vi "InterTrial.vi"(8 "error in (no error)":errorcluster, 11 "TrialBasedExperiment in":refnum<class "MatlabExperiment.lvclass">) -> (0 "error out":errorcluster, 2 "Timeout":dbl, 3 "TrialBasedExperiment out":refnum<class "MatlabExperiment.lvclass">)   [LabVIEW 2010, in "MatlabExperiment.lvclass"]
uses:
  MatlabExperiment.lvclass
  TrialBasedExperimentObject/TrialBasedExperiment.lvclass
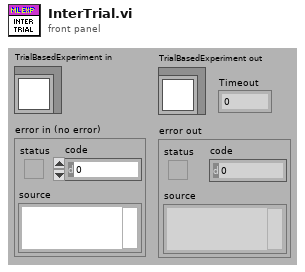
[diagram p1: front panel]
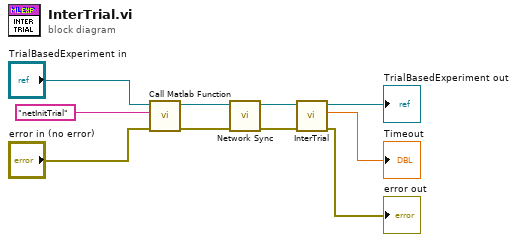
[diagram p0: block diagram]
diagram:
  n1 = call-dynamic "Call Matlab Function.vi"("error in (no error)"="error in (no error)", "Function name"="netInitTrial", "TrialBasedExperiment in"="TrialBasedExperiment in") -> ("error out"=w3:errorcluster, "TrialBasedExperiment out"=w4:refnum<class "MatlabExperiment.lvclass">)  [unwired: 5 in, 2 out]
  n2 = call "Network Sync.vi"("error in (no error)"=w3, "MatlabExperiment in"=w4) -> ("error out"=w2:errorcluster, "MatlabExperiment out"=w1:refnum<class "MatlabExperiment.lvclass">)  [unwired: 8 in]
  n3 = call-parent "InterTrial.vi"("error in (no error)"=w2, "TrialBasedExperiment in"=w1) -> ("error out"=→"error out":errorcluster, "Timeout"=→"Timeout":dbl, "TrialBasedExperiment out"=→"TrialBasedExperiment out":refnum<class "MatlabExperiment.lvclass">)  [unwired: 7 in]
